vi "MultiLOOPs Parallelism.vi"() -> ()   [LabVIEW 2020]
panel:
  out "Chart":dbl(graph)
  in  "PauseDAQ":bool
  in  "Exit":bool
  in  "StartDAQ":bool
  # "Messages will be sent\nto DAQ Loop to contol\nthe DAQ Start / Pause."
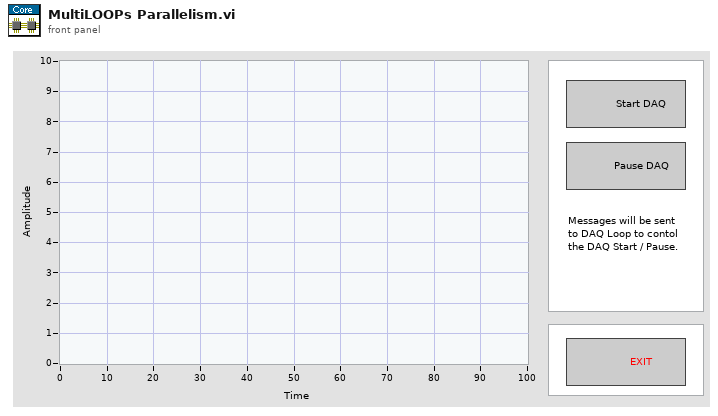
[diagram p1: front panel]
types:
  T1 = cluster{"UserEvent1":refnum<user-event>, "UserEvent2":refnum<user-event>}
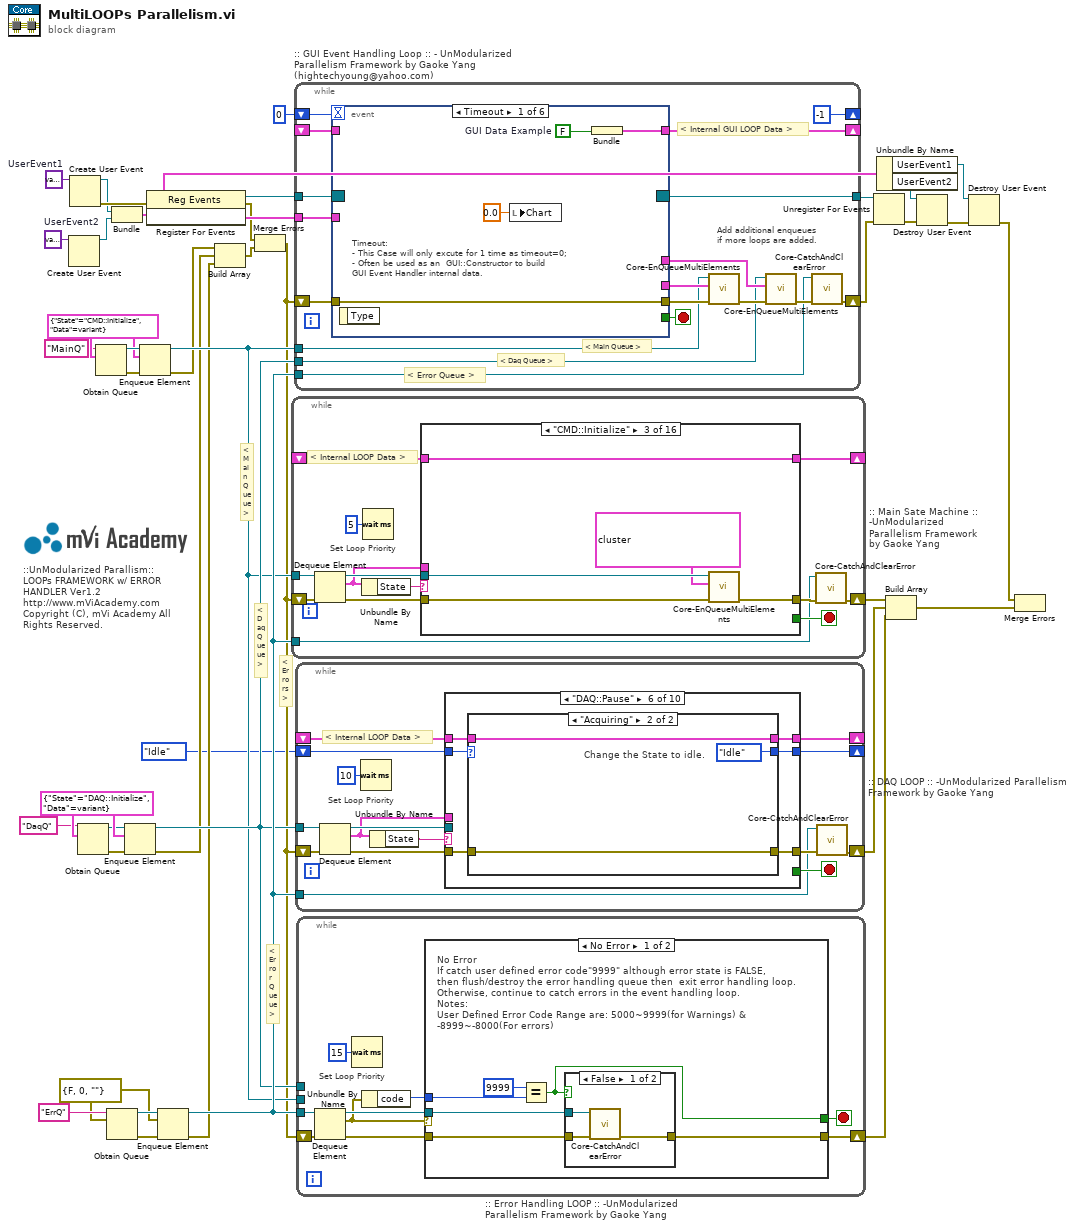
[diagram p0: block diagram]
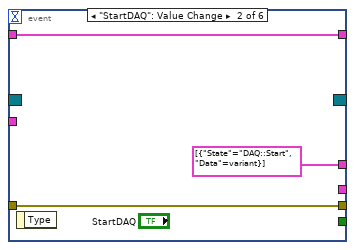
[diagram p2: hidden frame]
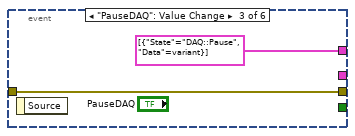
[diagram p3: hidden frame]
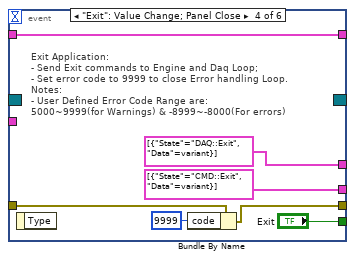
[diagram p4: hidden frame]
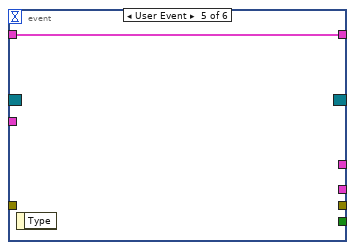
[diagram p5: hidden frame]
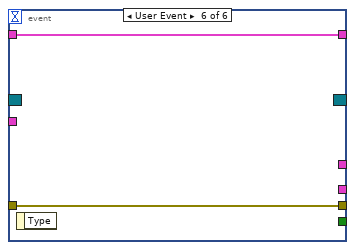
[diagram p6: hidden frame]
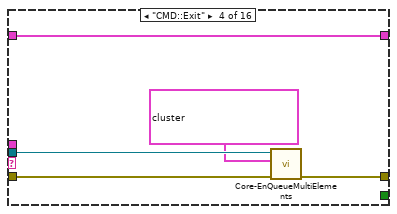
[diagram p9: hidden frame]
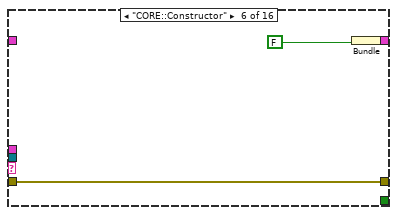
[diagram p11: hidden frame]
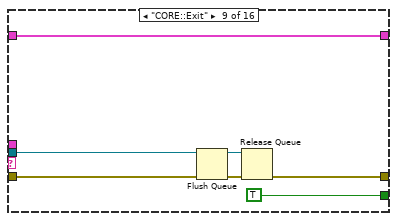
[diagram p14: hidden frame]
diagram:
  w16 = variant  # UserEvent2
  w20 = variant  # UserEvent1
  w30 = errorcluster {"status"=FALSE, "code"=0, "source"=""} ("error in (no error)")
  w37 = cluster{"State":string, "Data":variant} {"State"="DAQ::Initialize", "Data"=variant} ("DaqQueue")
  w39 = cluster{"State":string, "Data":variant} {"State"="CMD::Initialize", "Data"=variant} ("MainQueue")
  # "::UnModularized Parallism::\nLOOPs FRAMEWORK w/ ERROR HANDLER Ver1.2\nhttp://www.mViAcademy.com\nCopyright (C), mVi Academy All Rights Reserved."
  # "< Errors >"
  # "< Error Queue >"
  # "< Daq Queue >"
  # "< Main Queue >"
  n1 = Create User Event(user event datatype=w16) -> (user event=w14:refnum<user-event>)  [unwired: 1 in, 1 out]
  n2 = Create User Event(user event datatype=w20) -> (user event=w15:refnum<user-event>, error out=w19:errorcluster)  [unwired: 1 in]
  n3 = Obtain Queue(name (unnamed)="DaqQ", element data type=w37) -> (queue out=w35:refnum<queue>, error out=w36:errorcluster)  [unwired: 3 in, 1 out]
  n4 = Obtain Queue(name (unnamed)="MainQ", element data type=w39) -> (queue out=w41:refnum<queue>, error out=w40:errorcluster)  [unwired: 3 in, 1 out]
  n5 = Obtain Queue(name (unnamed)="ErrQ", element data type=w30) -> (queue out=w32:refnum<queue>, error out=w31:errorcluster)  [unwired: 3 in, 1 out]
  n6 = Bundle("UserEvent1"=w15, "UserEvent2"=w14) -> (w13:T1)  [unwired: 1 in]
  n7 = Enqueue Element(queue=w35, element=w37, error in (no error)=w36) -> (queue out=w23:refnum<queue>, error out=w3:errorcluster)  [unwired: 2 out]
  n8 = Enqueue Element(queue=w41, element=w39, error in (no error)=w40) -> (queue out=w22:refnum<queue>, error out=w4:errorcluster)  [unwired: 2 out]
  n9 = register-events(error in=w19, w13) -> (reference out=w8:refnum<event-registration>, error out=w2:errorcluster)  [unwired: 1 in]
  n10 = Enqueue Element(queue=w32, element=w30, error in (no error)=w31) -> (queue out=w28:refnum<queue>, error out=w5:errorcluster)  [unwired: 2 out]
  n11 = Build Array(w4, w3, w5) -> (w6:errorcluster[])
  n12 = Merge Errors(w2, w6) -> (w21:errorcluster)
  n13 = while ":: Main Sate Machine :: -UnModularized Parallelism Framework by Gaoke Yang" {
    tunnel: w22 -> [w54]
    shift-right: [w44] -> w26
    shift-left: w21 -> [w46]
    shift-right: [w48] -> _
    shift-left: _ -> [w47]
    tunnel: w28 -> [w43]
    stop <- w51 stop-if-true
    # "Set Loop Priority"
    # "< Internal LOOP Data >"
    n14 = Dequeue Element(queue=w54, error in (no error)=w46) -> (queue out=w52:refnum<queue>, element=w49:cluster{"State":string, "Data":variant}, error out=w53:errorcluster)  [unwired: 2 out]
    n15 = Unbundle By Name(w49) -> ("State"=w50:string)
    n16 = Wait (ms)(milliseconds to wait=u32 5) -> ()  [unwired: 1 out]
    n17 = case shown="\"CMD::Initialize\"" w50 {
      tunnel: [w55 w58 w62 w67 w70 w73 w75 w77 w80 w85 w87 w89 w92 w94 w96 w97] -> w45
      tunnel: [_ _ _ _ _ _ _ _ TRUE _ _ _ _ _ _ _] -> w51
      tunnel: w52 -> [_ _ w63 w66 _ _ _ _ w83 _ _ _ _ _ _ _]
      tunnel: w53 -> [w55 w58 w59 w68 w70 w73 w75 w77 w82 w85 w87 w89 w92 w94 w96 w97]
      tunnel: w49 -> [_ _ _ _ _ _ _ _ _ _ _ _ _ _ _ _]
      tunnel: [w56 w57 w60 w64 w69 w71 w74 w76 w78 w86 w88 w90 w91 w93 w95 w98] -> w48
      tunnel: w47 -> [w56 w57 w60 w64 w69 _ w74 w76 w78 w86 w88 w90 w91 w93 w95 w98]
      frame "IDLE", Default {
      }
      frame "-------- Commands ---------" {
      }
      frame "CMD::Initialize" {
        n18 = call "Core-EnQueueMultiElements.vi"("ErrorIn"=w59, "CmdArray"=cluster{"State":string, "Data":variant}[] [{"State"="CORE::Constructor", "Data"=variant}, {"State"="CORE::Initialize", "Data"=variant}], "QRefIn"=w63) -> ("ErrorOut"=w62:errorcluster)  [unwired: 8 in]
      }
      frame "CMD::Exit" {
        n19 = call "Core-EnQueueMultiElements.vi"("ErrorIn"=w68, "CmdArray"=cluster{"State":string, "Data":variant}[] [{"State"="CORE::DeConstructor", "Data"=variant}, {"State"="CORE::Exit", "Data"=variant}], "QRefIn"=w66) -> ("ErrorOut"=w67:errorcluster)  [unwired: 8 in]
      }
      frame "------------ Core ------------" {
      }
      frame "CORE::Constructor" {
        n20 = Bundle(FALSE) -> (w71:cluster{bool})  [unwired: 1 in]
      }
      frame "CORE::Initialize" {
      }
      frame "CORE::DeConstructor" {
      }
      frame "CORE::Exit" {
        n21 = Flush Queue(queue=w83, error in (no error)=w82) -> (queue out=w79:refnum<queue>, error out=w81:errorcluster)  [unwired: 1 out]
        n22 = Release Queue(queue=w79, error in (no error)=w81) -> (error out=w80:errorcluster)  [unwired: 1 in, 2 out]
      }
      frame "------------  GUI  -------------" {
      }
      frame "GUI::Initialize" {
      }
      frame "GUI::SetCusor" {
      }
      frame "GUI::SetMenu" {
      }
      frame "----------- USER -----------" {
      }
      frame "USER::Case1" {
      }
      frame "USER::Case2" {
      }
    }
    n23 = call "Core-CatchAndClearError.vi"("Err-I"=w45, "ErrQ-I"=w43) -> ("Err-O"=w44:errorcluster)  [unwired: 9 in]
  }
  n24 = while ":: GUI Event Handling Loop :: - UnModularized Parallelism Framework by Gaoke Yang (hightechyoung@yahoo.com)" {
    tunnel: w22 -> [w112]
    shift-right: [w106] -> w17
    shift-left: w21 -> [w116]
    tunnel: w23 -> [w109]
    tunnel: w28 -> [w107]
    shift-right: [-1] -> _
    shift-left: 0 -> [w104]
    shift-right: [w103] -> _
    shift-left: _ -> [w102]
    tunnel: w8 -> [w101]
    tunnel: w13 -> [w100]
    tunnel: [w99] -> w7
    stop <- w110 stop-if-true
    # "< Internal GUI LOOP Data >"
    # "Add additional enqueues \nif more loops are added."
    # "< Main Queue >"
    # "< Error Queue >"
    # "< Daq Queue >"
    n25 = event shown="[0] Timeout" {
      selector: w101 -> [_ _ _ _ _ _]
      dyn-events: [_ _ _ _ _ _] -> w99
      timeout: w104 -> [_ _ _ _ _ _]
      tunnel: [_ _ _ "Exit" _ _] -> w110
      tunnel: w116 -> [w120 w123 w124 w129 _ w134]
      tunnel: [w120 w123 w124 w128 _ w134] -> w114
      tunnel: [_ _ _ cluster{"State":string, "Data":variant}[] [{"State"="CMD::Exit", "Data"=variant}] _ _] -> w115
      tunnel: [_ cluster{"State":string, "Data":variant}[] [{"State"="DAQ::Start", "Data"=variant}] cluster{"State":string, "Data":variant}[] [{"State"="DAQ::Pause", "Data"=variant}] cluster{"State":string, "Data":variant}[] [{"State"="DAQ::Exit", "Data"=variant}] _ _] -> w111
      tunnel: [w118 w121 _ w126 w133 w135] -> w103
      tunnel: w102 -> [_ w121 _ w126 w133 w135]
      tunnel: w100 -> [_ _ _ _ _ _]
      event Timeout {
        w119 = FALSE  # GUI Data Example
        # "Timeout:\n- This Case will only excute for 1 time as timeout=0;\n- Often be used as an  GUI::Constructor to build\nGUI Event Handler internal data."
        n26 = event-data() -> ()  [unwired: 2 out]
        n27 = local write "Chart"(0.0 ("Chart")) -> ()
        n28 = Bundle("GUI Data Example"=w119) -> (w118:cluster{"GUI Data Example":bool})  [unwired: 1 in]
      }
      event "StartDAQ": Value Change {
        n29 = event-data() -> ()  [unwired: 2 out]
      }
      event "PauseDAQ": Value Change {
        n30 = event-data() -> ()  [unwired: 2 out]
      }
      event "Exit": Value Change; Panel Close {
        # "Exit Application:\n- Send Exit commands to Engine and Daq Loop;\n- Set error code to 9999 to close Error handling Loop.\nNotes:\n- User Defined Error Code Range are:\n5000~9999(for Warnings) & -8999~-8000(For errors)"
        n31 = event-data() -> ()  [unwired: 2 out]
        n32 = Bundle By Name(cluster=w129, "code"=9999) -> (w128:errorcluster)
      }
      event User Event {
        n33 = event-data() -> ()  [unwired: 2 out]
      }
      event User Event {
        n34 = event-data() -> ()  [unwired: 2 out]
      }
    }
    n35 = call "Core-EnQueueMultiElements.vi"("ErrorIn"=w114, "CmdArray"=w115, "QRefIn"=w112) -> ("ErrorOut"=w113:errorcluster)  [unwired: 8 in]
    n36 = call "Core-EnQueueMultiElements.vi"("ErrorIn"=w113, "CmdArray"=w111, "QRefIn"=w109) -> ("ErrorOut"=w108:errorcluster)  [unwired: 8 in]
    n37 = call "Core-CatchAndClearError.vi"("Err-I"=w108, "ErrQ-I"=w107) -> ("Err-O"=w106:errorcluster)  [unwired: 9 in]
  }
  n38 = while ":: DAQ LOOP :: -UnModularized Parallelism Framework by Gaoke Yang" {
    tunnel: w23 -> [w150]
    shift-right: [w139] -> w27
    shift-left: w21 -> [w145]
    shift-right: [w143] -> _
    shift-left: _ -> [w142]
    tunnel: w28 -> [w138]
    shift-right: [w136] -> _
    shift-left: enum16{"Idle", "Acquiring"}."Idle" -> [w137]
    stop <- w148 stop-if-true
    # "Set Loop Priority"
    # "< Internal LOOP Data >"
    n39 = Dequeue Element(queue=w150, error in (no error)=w145) -> (queue out=w147:refnum<queue>, element=w144:cluster{"State":string, "Data":variant}, error out=w149:errorcluster)  [unwired: 2 out]
    n40 = Wait (ms)(milliseconds to wait=u32 10) -> ()  [unwired: 1 out]
    n41 = Unbundle By Name(w144) -> ("State"=w146:string)
    n42 = case shown="\"DAQ::Pause\"" w146 {
      tunnel: w149 -> [w152 w156 w158 w164 w182 w201 w209 w217 w221 w224]
      tunnel: [w152 w156 w158 w163 w183 w200 w209 w214 w221 w224] -> w140
      tunnel: [_ _ _ _ _ _ _ TRUE _ _] -> w148
      tunnel: w147 -> [_ _ _ w165 w181 _ _ w216 _ _]
      tunnel: w144 -> [_ _ _ _ _ _ _ _ _ _]
      tunnel: [w153 w155 w159 w161 w177 w196 w210 w212 w220 w223] -> w143
      tunnel: w142 -> [w153 w155 _ w162 w178 w197 w210 w212 w220 w223]
      tunnel: w137 -> [w151 w154 w157 w167 w180 w199 w208 w211 w219 w222]
      tunnel: [w151 w154 w157 w166 w179 w198 w208 w211 w219 w222] -> w136
      frame "IDLE", Default {
      }
      frame "-------- DAQ ---------" {
      }
      frame "DAQ::Initialize" {
        n43 = Bundle(FALSE) -> (w159:cluster{bool})  [unwired: 1 in]
      }
      frame "DAQ::Start" {
        n44 = case shown="\"Idle\", Default" w167 {
          selector: w167 -> [_ w176]
          tunnel: [enum16{"Idle", "Acquiring"}."Acquiring" w176] -> w166
          tunnel: w165 -> [w171 _]
          tunnel: w164 -> [w170 w175]
          tunnel: [w169 w175] -> w163
          tunnel: w162 -> [w168 w174]
          tunnel: [w168 w174] -> w161
          frame "Idle", Default {
            n45 = Enqueue Element(queue=w171, element=cluster{"State":string, "Data":variant} {"State"="DAQ::Acquiring", "Data"=variant} ("DaqQueue"), error in (no error)=w170) -> (error out=w169:errorcluster)  [unwired: 3 out]
          }
          frame "Acquiring" {
            # "The system is already acquiring. \nIgnore the \"Start\" message."
          }
        }
      }
      frame "DAQ::Acquiring" {
        n46 = case shown="\"Acquiring\"" w180 {
          selector: w180 -> [w185 w188]
          tunnel: [w184 w195] -> w183
          tunnel: w182 -> [w184 w194]
          tunnel: w181 -> [_ w192]
          tunnel: [w185 w188] -> w179
          tunnel: w178 -> [w186 w187]
          tunnel: [w186 w187] -> w177
          frame "Idle", Default {
            # "Ignore \"Acquire\" command when the acquisition is idle."
          }
          frame "Acquiring" {
            n47 = Random Number (0-1)() -> (number: 0 to 1=w191:dbl)
            n48 = Multiply(x=w191, y=10.0) -> (x*y=→"Chart":dbl)
            n49 = Enqueue Element(queue=w192, element=cluster{"State":string, "Data":variant} {"State"="DAQ::Acquiring", "Data"=variant} ("DaqQueue"), error in (no error)=w194) -> (error out=w195:errorcluster)  [unwired: 3 out]
          }
        }
      }
      frame "DAQ::Pause" {
        n50 = case shown="\"Acquiring\"" w199 {
          selector: w199 -> [w202 _]
          tunnel: w201 -> [w204 w207]
          tunnel: [w204 w207] -> w200
          tunnel: [w202 enum16{"Idle", "Acquiring"}."Idle"] -> w198
          tunnel: w197 -> [w203 w205]
          tunnel: [w203 w205] -> w196
          frame "Idle", Default {
            # "Already idle, ignore Pause command."
          }
          frame "Acquiring" {
            # "Change the State to idle."
          }
        }
      }
      frame "DAQ::UnInitialize" {
      }
      frame "DAQ::Exit" {
        # "Close the device here."
        n51 = Flush Queue(queue=w216, error in (no error)=w217) -> (queue out=w213:refnum<queue>, error out=w215:errorcluster)  [unwired: 1 out]
        n52 = Release Queue(queue=w213, error in (no error)=w215) -> (error out=w214:errorcluster)  [unwired: 1 in, 2 out]
      }
      frame "--------User Case---------" {
      }
      frame "Reserved" {
      }
    }
    n53 = call "Core-CatchAndClearError.vi"("Err-I"=w140, "ErrQ-I"=w138) -> ("Err-O"=w139:errorcluster)  [unwired: 9 in]
  }
  n54 = while ":: Error Handling LOOP :: -UnModularized Parallelism Framework by Gaoke Yang" {
    tunnel: w28 -> [w233]
    shift-right: [w227] -> w25
    shift-left: w21 -> [w229]
    tunnel: w23 -> [_]
    tunnel: w22 -> [_]
    stop <- w231 stop-if-true
    # "Set Loop Priority"
    n55 = Dequeue Element(queue=w233, error in (no error)=w229) -> (queue out=w230:refnum<queue>, element=w228:errorcluster, error out=w232:errorcluster)  [unwired: 2 out]
    n56 = Wait (ms)(milliseconds to wait=u32 15) -> ()  [unwired: 1 out]
    n57 = Unbundle By Name(w228) -> ("code"=w226:i32)
    n58 = case shown="No Error" w228 {
      selector: w228 -> [_ w251]
      tunnel: w232 -> [w239 _]
      tunnel: [w238 w250] -> w227
      tunnel: [w236 w249] -> w231
      tunnel: w230 -> [w237 w248]
      tunnel: w226 -> [w235 w252]
      frame No Error {
        # "No Error\nIf catch user defined error code\"9999\" although error state is FALSE, \nthen flush/destroy the error handling queue then  exit error handling loop.\nOtherwise, continue to catch errors in the event handling loop.\nNotes:\nUser Defined Error Code Range are: 5000~9999(for Warnings) & -8999~-8000(For errors)"
        n59 = Equal?(x=9999, y=w235) -> (x = y?=w236:bool)
        n60 = case shown="False" w236 {
          tunnel: w239 -> [w241 w246]
          tunnel: [w240 w245] -> w238
          tunnel: w237 -> [w242 w244]
          frame False {
            n61 = call "Core-CatchAndClearError.vi"("Err-I"=w241, "ErrQ-I"=w242) -> ("Err-O"=w240:errorcluster)  [unwired: 9 in]
          }
          frame True {
            n62 = Flush Queue(queue=w244, error in (no error)=w246) -> (queue out=w247:refnum<queue>, error out=w243:errorcluster)  [unwired: 1 out]
            n63 = Release Queue(queue=w247, error in (no error)=w243) -> (error out=w245:errorcluster)  [unwired: 3 out]
          }
        }
      }
      frame Error {
        n64 = case shown="0, Default" w252 {
          tunnel: w251 -> [w255]
          tunnel: [errorcluster {"status"=FALSE, "code"=0, "source"=""} ("error out")] -> w250
          tunnel: [FALSE] -> w249
          tunnel: w248 -> [_]
          frame 0, Default {
            # "Error\nErrors will be throw here for handling.\nAdd error handling case and code if you want to handle specific error code.\nNotes:\n- You can use User Defined Error Code in your program;\n-  User Defined Error Code Range are: 5000~9999(for Warnings) & -8999~-8000(For errors)"
            n65 = call <vilib>:"General Error Handler.vi"("[user-defined codes]"=i32[] [9998], "[user-defined descriptions]"=string[] ["USER Error!"], "error in (no error)"=w255) -> ()  [unwired: 8 in, 5 out]
          }
        }
      }
    }
  }
  n66 = Unregister For Events(event registration refnum=w7, error in=w17) -> (error out=w18:errorcluster)
  n67 = Unbundle By Name(w13) -> ("UserEvent1"=w11:refnum<user-event>, "UserEvent2"=w12:refnum<user-event>)
  n68 = Build Array(w26, w27, w25) -> (w24:errorcluster[])
  n69 = Destroy User Event(user event=w12, error in=w18) -> (error out=w10:errorcluster)
  n70 = Destroy User Event(user event=w11, error in=w10) -> (error out=w9:errorcluster)
  n71 = Merge Errors(w9, w24) -> ()  [unwired: 1 out]
